vi "Create Engine Folder and Copy RT Template.vi"(8 "error in (no error)":errorcluster, 9 "Project Root":path, 10 "Project Name":string, 11 "CD Template":refnum<class "NIVS_CD Template.lvclass">) -> (0 "error out":errorcluster)   [LabVIEW 2015, in "NIVS_CD Template.lvclass"]
uses:
  NIVS_CD Template.lvclass
  NIVS_Consolidated_CDW_MetaDataObj/CD Engine lvlib.ctl
  NIVS_Consolidated_CDW_MetaDataObj/NIVS_Consolidated_CDW_MetaDataObj.lvclass
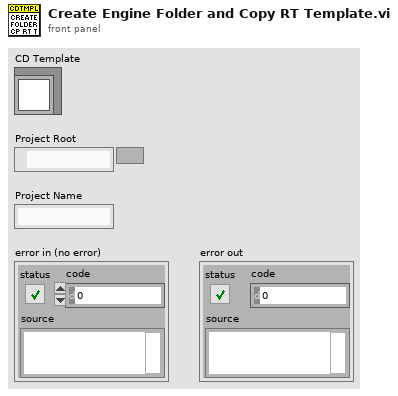
[diagram p1: front panel]
types:
  T1 = typedef "NIVS_Consolidated_CDW_MetaDataObj.lvclass/CD Engine lvlib.ctl" = enum16{"LibraryFileName", "LibraryFolderName", "Engine.FolderName", "Engine.Init.FolderName", "Engine.Run.FolderName", "Engine.Shutdown.FolderName", "Types.FolderName", "Engine.RT Driver VI.TemplatePath", "Engine.RT Driver VI.FileName", "Engine.RTStateVariables.Name", "Engine.RTStateVariables.Name.NoExtension", "Engine.Async.NameExtension", "Engine.Async.TemplateName"}
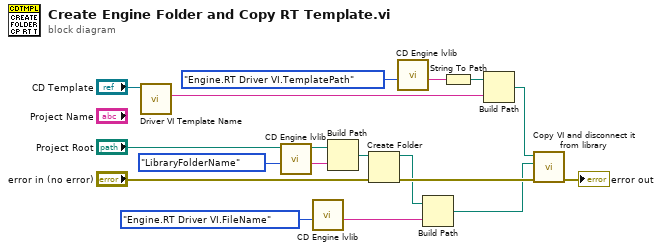
[diagram p0: block diagram]
diagram:
  n1 = call-dynamic "Driver VI Template Name.vi"("CD Template"="CD Template") -> ("Driver VI Template Name"=w1:string)  [unwired: 10 in]
  n2 = call "CD Engine lvlib.vi"("Action"=CD_Engine_lvlib."LibraryFolderName") -> ("Output"=w4:string)  [unwired: 10 in]
  n3 = call "CD Engine lvlib.vi"("Action"=CD_Engine_lvlib."Engine.RT Driver VI.FileName") -> ("Output"=w6:string)  [unwired: 10 in]
  n4 = Build Path(base path="Project Root", name or relative path=w4) -> (appended path=w3:path)
  n5 = Create Folder(path (use dialog)=w3, error in="error in (no error)") -> (created path=w5:path, error out=w17:errorcluster)  [unwired: 1 in, 1 out]
  n6 = call "CD Engine lvlib.vi"("Action"=CD_Engine_lvlib."Engine.RT Driver VI.TemplatePath") -> ("Output"=w8:string)  [unwired: 10 in]
  n7 = Build Path(base path=w5, name or relative path=w6) -> (appended path=w7:path)
  n8 = String To Path(string=w8) -> (path=w9:path)
  n9 = Build Path(base path=w9, name or relative path=w1) -> (appended path=w10:path)
  n10 = call "Copy VI and disconnect it from library.vi"("error in (no error)"=w17, "VI Target Path"=w7, "VI Source Path"=w10) -> ("error out"=→"error out":errorcluster)  [unwired: 8 in]
